vi "Step3_Touch.vi"   [LabVIEW 2012]
uses:
  <vilib>/NXT/Subs/MotorOutput.ctl
  <vilib>/NXT/Block Support/NXT_InputPort.ctl
types:
  T1 = typedef "MotorOutput.ctl" = u8
  T2 = typedef "NXT_InputPort.ctl" = u32
  T3 = typedef "LVHSConnector.ctl" = refnum<class "BrickReference.lvclass">
  T4 = typedef "ColorSensorColors.ctl" = enum16{"No Color", "Black", "Blue", "Green", "Yellow", "Red", "White", "Brown"}
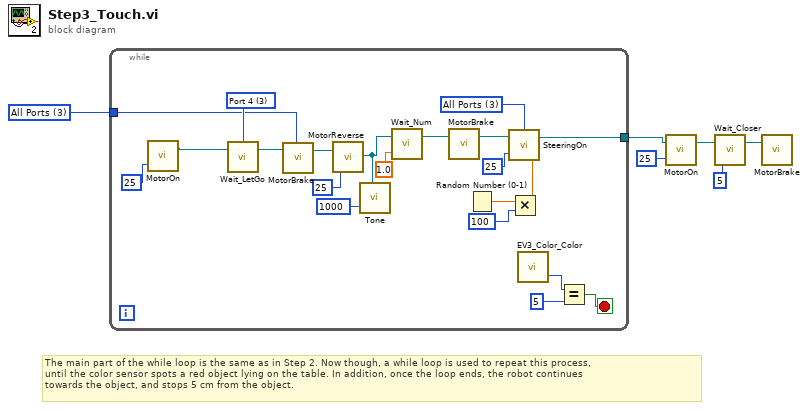
[diagram p0: block diagram]
diagram:
  w6 = T1 3 items=["Port A"=0, "Port B"=1, "Port C"=2, "Ports A & B"=4, "Ports A & C"=5, "Ports B & C"=6, "All Ports"=3] ("Output Port (All Ports)")
  # "The main part of the while loop is the same as in Step 2. Now though, a while loop is used to repeat this process,\nuntil the color sensor spots a red object lying on the table. In addition, once the loop ends, the robot continues \ntowards the object, and stops 5 cm from the object."
  n1 = while {
    tunnel: w6 -> [w25]
    tunnel: [w9] -> w5
    stop <- w10 stop-if-true
    w20 = T1 3 items=["Port A"=0, "Port B"=1, "Port C"=2, "Ports A & B"=4, "Ports A & C"=5, "Ports B & C"=6, "All Ports"=3] ("Output Ports (A & B)")
    w27 = T2 3 items=["Port 1", "Port 2", "Port 3", "Port 4"] ("Port (Port 1)")
    n2 = call <vilib>:"MotorOn.vi"("Power (75)"=25) -> ("NXT/EV3"=w17:T3)  [unwired: 3 in]
    n3 = call <vilib>:"Wait_LetGo.vi"("NXT/EV3"=w17, "Port (Port 1)"=w27) -> ("NXTEV3"=w26:T3)  [unwired: 2 in]
    n4 = call <vilib>:"MotorBrake.vi"("NXT/EV3"=w26, "Port (All Ports)"=w25) -> ("NXT/EV3"=w24:T3)  [unwired: 2 in]
    n5 = call <vilib>:"MotorReverse.vi"("Power (75)"=25, "NXT/EV3"=w24) -> ("NXT/EV3"=w23:T3)  [unwired: 2 in]
    n6 = call <vilib>:"Tone.vi"("Duration (500 ms)"=u16 1000, "NXT/EV3"=w23) -> ()  [unwired: 2 in, 1 out]
    n7 = call <vilib>:"Wait_Num.vi"("Time (1 sec)"=sgl 1.0, "NXT/EV3"=w23) -> ("NXT/EV3"=w22:T3)  [unwired: 2 in]
    n8 = call <vilib>:"MotorBrake.vi"("NXT/EV3"=w22) -> ("NXT/EV3"=w21:T3)  [unwired: 3 in]
    n9 = Random Number (0-1)() -> (number: 0 to 1=w15:dbl)
    n10 = Multiply(x=w15, y=100) -> (x*y=w13:dbl)
    n11 = call <vilib>:"SteeringOn.vi"("Power (75)"=25, "Steering (100)"=w13, "NXT/EV3"=w21, "Output Ports (A & B)"=w20) -> ("NXT/EV3"=w9:T3)
    n12 = call <vilib>:"EV3_Color_Color.vi"() -> ("Detected Color"=w11:T4)  [unwired: 3 in, 1 out]
    n13 = Equal?(x=w11, y=5) -> (x = y?=w10:bool)
  }
  n14 = call <vilib>:"MotorOn.vi"("Power (75)"=25, "NXT/EV3"=w5) -> ("NXT/EV3"=w3:T3)  [unwired: 2 in]
  n15 = call <vilib>:"Wait_Closer.vi"("Distance (40)"=i16 5, "NXT/EV3"=w3) -> ("NXT/EV3"=w1:T3)  [unwired: 2 in]
  n16 = call <vilib>:"MotorBrake.vi"("NXT/EV3"=w1) -> ()  [unwired: 3 in, 1 out]
